vi "Worker List Menu Selection.vi"(8 "error in (no error)":errorcluster, 9 "Menu Item Tag":string, 10 "Worker Name":string, 11 "BuildServer in":refnum<class "BuildServer.lvclass">) -> (0 "error out":errorcluster, 3 "BuildServer out":refnum<class "BuildServer.lvclass">)   [LabVIEW 2017, in "BuildServer.lvlib" / "BuildServer.lvclass"]
uses:
  BuildServer.lvclass
  BuildServer.lvclass/BuildServer.ctl
  Classes/Comm Interface/Comm Interface.lvclass
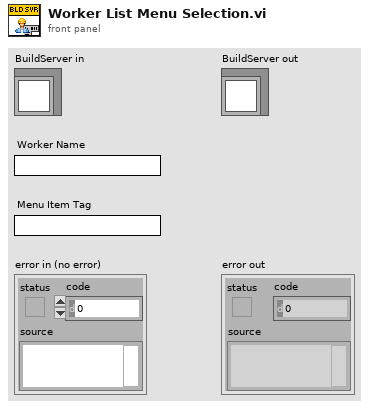
[diagram p1: front panel]
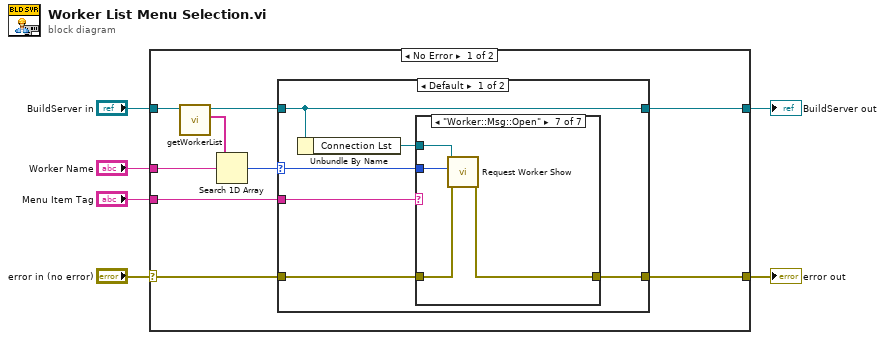
[diagram p0: block diagram]
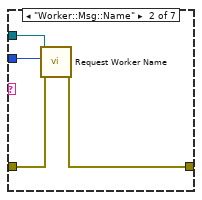
[diagram p3: hidden frame]
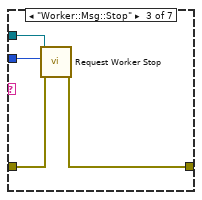
[diagram p4: hidden frame]
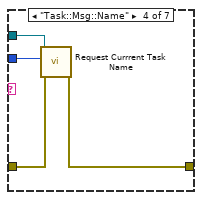
[diagram p5: hidden frame]
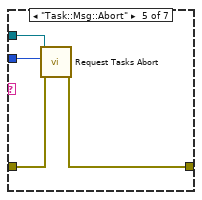
[diagram p6: hidden frame]
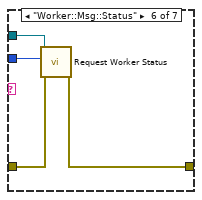
[diagram p7: hidden frame]
diagram:
  n1 = case shown="No Error" "error in (no error)" {
    selector: "error in (no error)" -> [w9 w49]
    tunnel: [w8 w49] -> w6
    tunnel: [w11 w50] -> w4
    tunnel: "BuildServer in" -> [w15 w50]
    tunnel: "Worker Name" -> [w13 _]
    tunnel: "Menu Item Tag" -> [w10 _]
    frame No Error {
      n2 = call "getWorkerList.vi"("BuildServer in"=w15) -> ("Worker List"=w14:string[], "BuildServer out"=w12:refnum<class "BuildServer.lvclass">)  [unwired: 8 in, 1 out]
      n3 = Search 1D Array(1D array=w14, element=w13) -> (index of element=w7:i32)  [unwired: 1 in]
      n4 = case shown="Default" w7 {
        selector: w7 -> [w19 _]
        tunnel: w12 -> [w21 w48]
        tunnel: [w21 w48] -> w11
        tunnel: w10 -> [w18 _]
        tunnel: w9 -> [w17 w47]
        tunnel: [w16 w47] -> w8
        frame Default {
          n5 = Unbundle By Name(w21) -> ("Connection Lst"=w20:refnum<class "Comm Interface.lvclass">)
          n6 = case shown="\"Worker::Msg::Open\"" w18 {
            tunnel: w20 -> [_ w26 w30 w34 w38 w42 w46]
            tunnel: w19 -> [_ w25 w29 w33 w37 w41 w45]
            tunnel: w17 -> [w22 w24 w28 w32 w36 w40 w44]
            tunnel: [w22 w23 w27 w31 w35 w39 w43] -> w16
            frame Default {
            }
            frame "Worker::Msg::Name" {
              n7 = call "Request Worker Name.vi"("error in (no error)"=w24, "index"=w25, "Comm Interface in"=w26) -> ("error out"=w23:errorcluster)  [unwired: 7 in, 1 out]
            }
            frame "Worker::Msg::Stop" {
              n8 = call "Request Worker Stop.vi"("error in (no error)"=w28, "index"=w29, "Comm Interface in"=w30) -> ("error out"=w27:errorcluster)  [unwired: 7 in, 1 out]
            }
            frame "Task::Msg::Name" {
              n9 = call "Request Currrent Task Name.vi"("error in (no error)"=w32, "index"=w33, "Comm Interface in"=w34) -> ("error out"=w31:errorcluster)  [unwired: 7 in, 1 out]
            }
            frame "Task::Msg::Abort" {
              n10 = call "Request Tasks Abort.vi"("error in (no error)"=w36, "index"=w37, "Comm Interface in"=w38) -> ("error out"=w35:errorcluster)  [unwired: 7 in, 1 out]
            }
            frame "Worker::Msg::Status" {
              n11 = call "Request Worker Status.vi"("error in (no error)"=w40, "index"=w41, "Comm Interface in"=w42) -> ("error out"=w39:errorcluster)  [unwired: 7 in, 1 out]
            }
            frame "Worker::Msg::Open" {
              n12 = call "Request Worker Show.vi"("error in (no error)"=w44, "index"=w45, "Comm Interface in"=w46) -> ("error out"=w43:errorcluster)  [unwired: 7 in, 1 out]
            }
          }
        }
        frame -1 {
        }
      }
    }
    frame Error {
    }
  }
  "error out" <- w6
  "BuildServer out" <- w4
